vi "updateValues.vi"(7 "Array of Device Number":i8[](array[numeric]), 8 "error in (no error)":errorcluster, 9 "channel index":i8, 10 "Array of Microsteps":dbl[](array[numeric]), 11 "VISA resource name":refnum<visa-resource-name>) -> (0 "error out":errorcluster, 3 "VISA resource name out":refnum<visa-resource-name>)   [LabVIEW 2020]
panel:
  out "Response String Array":string[](array[string])
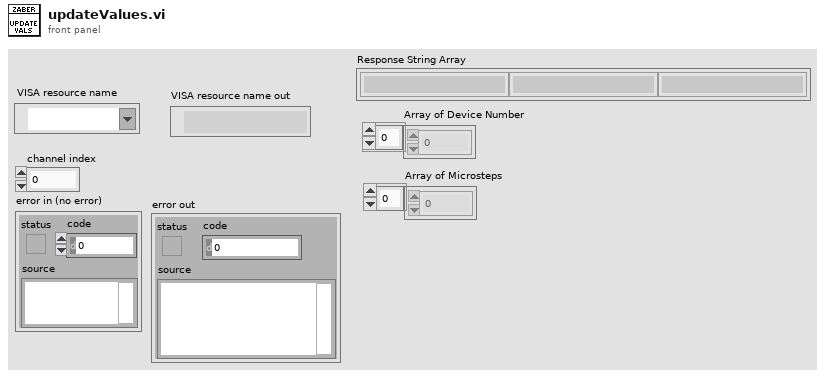
[diagram p1: front panel]
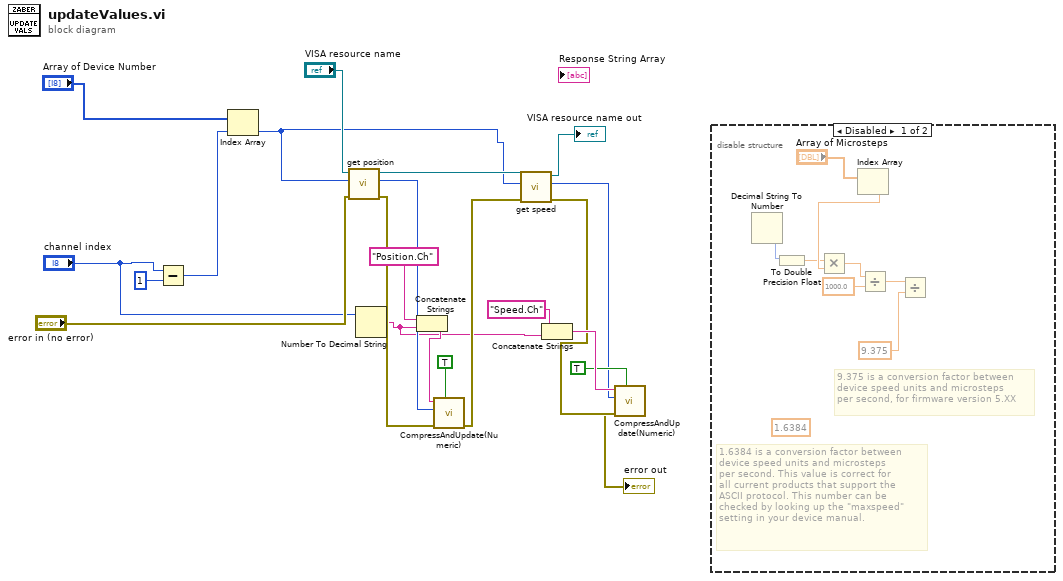
[diagram p0: block diagram]
diagram:
  n1 = Subtract(x="channel index", y=1) -> (x-y=w13:i32)
  n2 = Index Array(array="Array of Device Number", index=w13) -> (element=w3:i8)
  n3 = call "get position.vi"("error in (no error)"="error in (no error)", "Device Number"=w3, "VISA resource name"="VISA resource name") -> ("error out"=w17:errorcluster, "Data"=w16:i32, "VISA resource name out"=w4:refnum<visa-resource-name>)  [unwired: 5 in]
  n4 = Number To Decimal String(number="channel index") -> (decimal integer string=w7:string)  [unwired: 1 in]
  n5 = Concatenate Strings("Position.Ch" ("command or variable name"), w7) -> (w22:string)
  n6 = call "CompressAndUpdate(Numeric).vi"("force CVT update (false)"=TRUE, "error in"=w17, "Numeric"=w16, "command or variable name"=w22) -> ("error out"=w11:errorcluster)  [unwired: 7 in]
  n7 = call "get speed.vi"("error in (no error)"=w11, "Device Number"=w3, "VISA resource name"=w4) -> ("error out"=w6:errorcluster, "Data"=w1:i32, "VISA resource name out"=→"VISA resource name out":refnum<visa-resource-name>)  [unwired: 6 in]
  n8 = Concatenate Strings("Speed.Ch" ("command or variable name"), w7) -> (w10:string)
  n9 = call "CompressAndUpdate(Numeric).vi"("force CVT update (false)"=TRUE, "error in"=w6, "Numeric"=w1, "command or variable name"=w10) -> ("error out"=→"error out":errorcluster)  [unwired: 7 in]
  n10 = disable-structure shown="Disabled" {
    frame Disabled {
      (unwired) 1.6384 ("Speed Constant (1.6384)")
      # "9.375 is a conversion factor between \ndevice speed units and microsteps \nper second, for firmware version 5.XX"
      # "1.6384 is a conversion factor between \ndevice speed units and microsteps \nper second. This value is correct for\nall current products that support the\nASCII protocol. This number can be \nchecked by looking up the \"maxspeed\"\nsetting in your device manual."
      n11 = Decimal String To Number() -> (number=w29:i32)  [unwired: 3 in, 1 out]
      n12 = To Double Precision Float(number=w29) -> (double precision float=w27:dbl)
      n13 = Index Array(array="Array of Microsteps") -> (element=w28:dbl)  [unwired: 1 in]
      n14 = Multiply(x=w27, y=w28) -> (x*y=w26:dbl)
      n15 = Divide(x=w26, y=1000.0) -> (x/y=w24:dbl)
      n16 = Divide(x=w24, y=9.375 ("Speed Constant (1.6384)")) -> ()  [unwired: 1 out]
    }
    frame Enabled {
    }
  }
